vi "kCoerceFloat.vi"(8 "lower":dbl, 9 "input":dbl, 10 "upper":dbl) -> (0 "coerced?":bool, 2 "output":dbl)   [LabVIEW 2010, in "kevLib2010.lvlib"]
uses:
  kevLib2010.lvlib
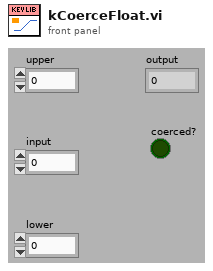
[diagram p1: front panel]
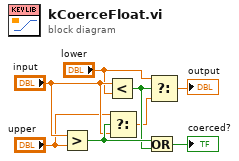
[diagram p0: block diagram]
diagram:
  n1 = Greater?(x="input", y="upper") -> (0:w7:bool)
  n2 = Less?(x="input", y="lower") -> (x < y?=w6:bool)
  n3 = Select(t="upper", s=w7, f="input") -> (s? t:f=w3:dbl)
  n4 = Or(x=w7, y=w6) -> (x .or. y?=→"coerced?":bool)
  n5 = Select(t="lower", s=w6, f=w3) -> (s? t:f=→"output":dbl)
